vi "Shutdown.vi"(8 "error in (no error)":errorcluster, 9 "TempQ in":refnum<queue>, 10 "ScanQ in":refnum<queue>, 11 "MaqQ in":refnum<queue>) -> (0 "error out":errorcluster, 1 "TempQ Out":refnum<queue>, 2 "ScanQ out":refnum<queue>, 3 "Queue out":refnum<queue>, 5 "Boolean":bool)   [LabVIEW 2025]
uses:
  Mag & Temp STM/CTLS/PSU Status.ctl
  Mag & Temp STM/CTLS/Scan_Params (QMH).ctl
  Downloads/OneDrive_2025-09-03/Instrument Controls/Temp Cntrl.ctl
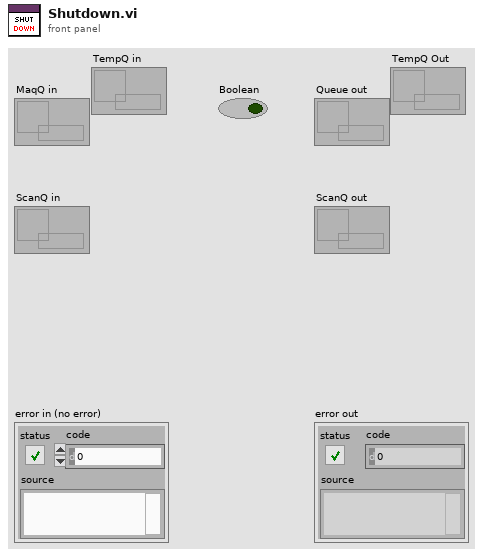
[diagram p1: front panel]
types:
  T1 = enum16{"1. INIT TEMP", "2. TC ON", "3. POLL_TEMPS", "4. TEMP_STAB", "5. TC IDLE", "6. APPLY NEXT TEMP", "7. TC OFF (Reset)"}
  T2 = typedef "Temp Cntrl.ctl" = cluster{"Range (0:Off)":u16, "Manual Output (0.00 %)":dbl, "Rate (D) (0.0 %)":dbl, "Reset (I) (20.0)":dbl, "Gain (P) (50.0)":dbl, "Power Up Enable (F: Disable)":bool, "Max User Current (2.000)":dbl, "Heater Resistance (1:25 Ohms)":u16, "Max Current (0:User Specified)":u16, "Heater Out Display (1:Current)":u16, "Mode (0:Off)":u16, "Input (0:None)":u16, "Target Temp (K)":dbl, "Serial Configuration":cluster{"Baud Rate":u32, "Parity":u16, "Data Bits":u16, "Stop Bits":u16, "Flow Control":u16}, "VISA resource name":refnum<visa-resource-name>, "Configure Control Parameters (0: Configure)":u16, "Enable Setpoint (F:Disable)":bool, "Input (0:A)":u16, "Data Source (0:Kelvin)":u16, "Output's Control Loop (1:1)":u16, "STND DEV Threshold ":dbl, "Mean Tolerance ":dbl, "Current State":enum16{"1. INIT TEMP", "2. TC ON", "3. POLL_TEMPS", "4. TEMP_STAB", "5. TC IDLE", "6. APPLY NEXT TEMP", "7. TC OFF (Reset)"}}
  T3 = enum16{"1. BIAS", "2. INIT_SCAN", "3. SCAN_IDLE", "4. INTER_SCAN", "5. NEW_COORDS_&_FRAME", "6. FINAL_SCAN", "7. POLL BIAS ", "8. Z-CONT.", "9. STOP"}
  T4 = typedef "Scan_Params (QMH).ctl" = cluster{"Setpoint (I)":dbl[], "Bias (V)":dbl[], "Number of scans":u8, "Port number (3364)":u32, "Avoid zero threshold (V)":dbl, "Current State":enum16{"1. BIAS", "2. POLL BIAS", "3. SCAN", "4. SCAN_IDLE", "5. Drift_Correct (SF)", "6. Drift_Correct (BS)", "7. STOP"}}
  T5 = enum16{"1. INIT MAG", "2. MAG ON", "3. MAG_STAB", "4. MAG IDLE", "5. PREP NEXT FIELD", "6. APPLY NEXT FIELD", "7. PREP OFF", "8. MAG OFF (Reset)"}
  T6 = typedef "PSU Status.ctl" = cluster{"Ramp Target":enum16{"ZERO", "MID", "MAX"}, "Pause":bool, "Switch Heater":bool, "Persistent Field":dbl, "Persistent Current":dbl, "Tesla":bool, "Output (T)":dbl, "Output (A)":dbl, "X Trip":enum16{"DISABLED", "ENABLED", "ACTIVE"}, "Ramp Rate (A/s)":dbl, "V Limit (V)":dbl, "Heater Voltage":dbl, "MAX Setpoint (A)":dbl, "MAX Setpoint (T)":dbl, "MID Setpoint (A)":dbl, "MID Setpoint (T)":dbl, "Lock":bool, "Field Constant":dbl, "Remote":bool, "Direction":enum16{"POSITIVE", "NEGATIVE", "OPEN", "UNIPOLAR"}, "Helium Level":u16, "Quench !":bool, "Voltage":dbl, "V Limit !":bool, "Ramping":bool, "At Target":bool, "Trip Field":dbl, "Trip Current":dbl, "Current State":enum16{"1. INIT MAG", "2. MAG ON", "3. MAG_STAB", "4. MAG IDLE", "5. MAG OFF (Reset)"}, "MAG Reference":refnum<visa-resource-name>}
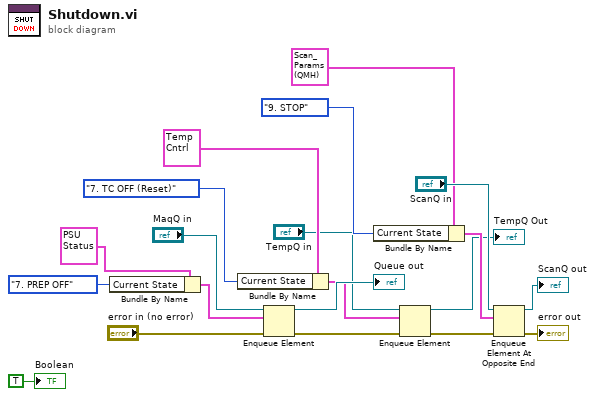
[diagram p0: block diagram]
diagram:
  n1 = Bundle By Name(cluster=T6 {"Ramp Target"=enum."ZERO", "Pause"=FALSE, "Switch Heater"=FALSE, "Persistent Field"=0.0, "Persistent Current"=0.0, "Tesla"=FALSE, "Output (T)"=0.0, "Output (A)"=0.0, "X Trip"=enum."DISABLED", "Ramp Rate (A/s)"=0.0, "V Limit (V)"=0.0, "Heater Voltage"=0.0, "MAX Setpoint (A)"=0.0, "MAX Setpoint (T)"=0.0, "MID Setpoint (A)"=0.0, "MID Setpoint (T)"=0.0, "Lock"=FALSE, "Field Constant"=0.0, "Remote"=FALSE, "Direction"=enum."POSITIVE", "Helium Level"=0, "Quench !"=FALSE, "Voltage"=0.0, "V Limit !"=FALSE, "Ramping"=FALSE, "At Target"=FALSE, "Trip Field"=0.0, "Trip Current"=0.0, "Current State"=enum."1. INIT MAG", "MAG Reference"="COM4"} ("PSU Status In"), "Current State"=T5."7. PREP OFF") -> (w12:T6)
  n2 = Bundle By Name(cluster=T2 {"Range (0:Off)"=0, "Manual Output (0.00 %)"=0.0, "Rate (D) (0.0 %)"=0.0, "Reset (I) (20.0)"=20.0, "Gain (P) (50.0)"=50.0, "Power Up Enable (F: Disable)"=FALSE, "Max User Current (2.000)"=2.0, "Heater Resistance (1:25 Ohms)"=1, "Max Current (0:User Specified)"=0, "Heater Out Display (1:Current)"=1, "Mode (0:Off)"=1, "Input (0:None)"=4, "Target Temp (K)"=5.0, "Serial Configuration"={"Baud Rate"=57600, "Parity"=1, "Data Bits"=7, "Stop Bits"=10, "Flow Control"=0}, "VISA resource name"="", "Configure Control Parameters (0: Configure)"=0, "Enable Setpoint (F:Disable)"=FALSE, "Input (0:A)"=3, "Data Source (0:Kelvin)"=0, "Output's Control Loop (1:1)"=2, "STND DEV Threshold "=0.1, "Mean Tolerance "=0.02, "Current State"=enum."1. INIT TEMP"} ("element"), "Current State"=T1."7. TC OFF (Reset)") -> (w3:T2)
  n3 = Enqueue Element(queue="MaqQ in", element=w12, error in (no error)="error in (no error)") -> (queue out=→"Queue out":refnum<queue>, error out=w19:errorcluster)  [unwired: 1 in, 1 out]
  n4 = Bundle By Name(cluster=T4 {"Setpoint (I)"=[], "Bias (V)"=[], "Number of scans"=1, "Port number (3364)"=3364, "Avoid zero threshold (V)"=0.004999999888241291, "Current State"=enum."1. BIAS"} ("element"), "Current State"=T3."9. STOP") -> (w16:T4)
  n5 = Enqueue Element(queue="TempQ in", element=w3, error in (no error)=w19) -> (queue out=→"TempQ Out":refnum<queue>, error out=w20:errorcluster)  [unwired: 1 in, 1 out]
  n6 = Enqueue Element At Opposite End(queue="ScanQ in", element=w16, error in (no error)=w20) -> (queue out=→"ScanQ out":refnum<queue>, error out=→"error out":errorcluster)  [unwired: 1 in, 1 out]
  "Boolean" <- TRUE
